vi "LegendWaveformGraph.vi"(7 "WaveformGraph in":refnum<vi>, 8 "error in (no error)":errorcluster, 9 "Plot.Visible":bool, 10 "Plot.Plot Name":string, 11 "Active Plot":i32) -> (0 "error out":errorcluster, 1 "Plot.Visible":bool, 2 "Plot.Plot Name":string, 3 "Active Plot":u32)   [LabVIEW 2016]
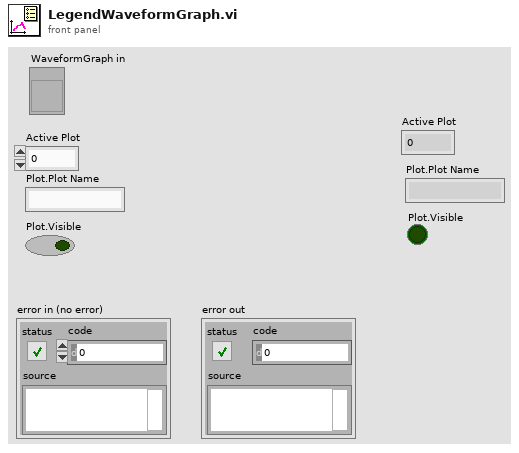
[diagram p1: front panel]
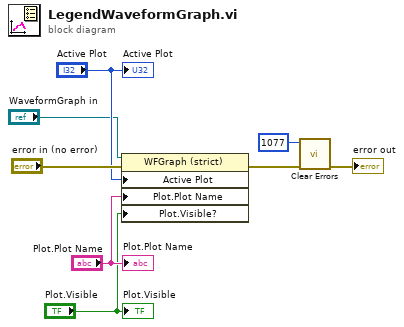
[diagram p0: block diagram]
diagram:
  n1 = property on="Property Node" class="WFGraph (strict)"(reference="WaveformGraph in", error in="error in (no error)", "Active Plot"="Active Plot", "Plot.Plot Name"="Plot.Plot Name", "Plot.Visible?"="Plot.Visible") -> (error out=w7:errorcluster)  [unwired: 1 out]
  n2 = call <vilib>:"Clear Errors.vi"("error in (no error)"=w7, "specific error code to clear (0: all)"=1077) -> ("error out"=→"error out":errorcluster)  [unwired: 4 in, 1 out]
  "Active Plot" <- "Active Plot"
  "Plot.Plot Name" <- "Plot.Plot Name"
  "Plot.Visible" <- "Plot.Visible"
